vi "Get Running.vi"(8 "error in (no error)":errorcluster, 11 "Panel in":refnum<class "Panel.lvclass">) -> (0 "error out":errorcluster, 2 "Running":bool, 3 "Panel out":refnum<class "Panel.lvclass">)   [LabVIEW 2018, in "OOPanel.lvlib" / "Panel.lvclass"]
uses:
  Panel.lvclass
  Panel.lvclass/Panel.ctl
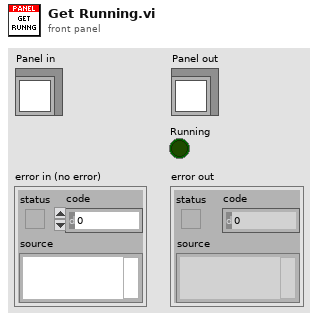
[diagram p1: front panel]
types:
  T1 = typedef "OOPanel.lvlib/Panel.lvclass/Ref Data.ctl" = cluster{"Panel VI":refnum<vi>, "Close":bool, "Panel Events":T2, "Running":bool, "Desired Size":T3, "Subpanel":refnum<vi>, "State":T4}
  T2 = typedef "OOPanel.lvlib/Panel.lvclass/Panel Events.ctl" = cluster{"Close":refnum<user-event>, "Visibility Changed":refnum<user-event>}
  T3 = typedef "OOPanel.lvlib/Panel.lvclass/Desired Size.ctl" = cluster{"Width":i16, "Height":i16}
  T4 = typedef "OOPanel.lvlib/Panel.lvclass/State.ctl" = enum16{"Idle", "Hidden", "Visible", "Subpanel"}
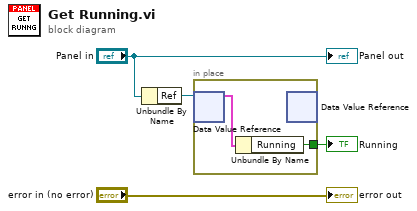
[diagram p0: block diagram]
diagram:
  n1 = Unbundle By Name("Panel in") -> ("Ref"=w3:refnum<data-value>)
  n2 = in-place {
    in-place-border: [w5] -> w1
    n3 = in-place-dvr #1(w3) -> (w6:T1)  [unwired: 1 out]
    n4 = Unbundle By Name(w6) -> ("Running"=w5:bool)
    n5 = in-place-dvr #1() -> ()  [unwired: 1 in, 2 out]
  }
  "Running" <- w1
  "error out" <- "error in (no error)"
  "Panel out" <- "Panel in"
